vi "JSON Difference.vi"() -> ()   [LabVIEW 2019]
doc: "Shows the use of JSON Difference in JSONtext."
uses:
  vi.lib/JDP Science/JSONtext/JSONtext.lvlib
panel:
  in  "Second":string="{\n    \"balance\": \"$3,124.10\",\n    \"index\": 1,\n    \"guid\": \"787c1912-662d-48b9-b395-2ad75d217224\",\n    \"isActive\": true,\n    \"_id\": \"59b53bcb02b0cb1b19bb98a8\",\n    \"latitude\": -14.331614,\n    \"longitude\": -65.032248,\n    \"tags\": [\n      \"sint\",\n      \"magna\",\n      \"laboris\",\n      \"irure\",\n      \"aliquip\",\n      \"voluptate\"\n    ],\n    \"picture\": \"http://placehold.it/32x32\",\n    \"age\": 28,\n    \"eyeColor\": \"green\",\n    \"name\": \"Brady York\",\n    \"gender\": \"male\",\n    \"company\": \"ELEMANTRA\",\n    \"email\": \"bradyyork@elemantra.com\",\n    \"phone\": \"+1 (932) 487-3511\",\n    \"address\": \"349 Amber Street, Day, Rhode Island, 8815\",\n    \"about\": \"Culpa magna magna incididunt aliquip adipisicing incididunt. Culpa ex qui aliqua aliqua sint aliqua incididunt duis. Labore consectetur in pariatur qui anim reprehenderit duis.\\r\\n\",\n    \"registered\": \"2014-10-21T08:11:24 -01:00\",\n    \"friends\": [\n      {\n        \"id\": 0,\n        \"name\": \"Magdalena Stanley\"\n      },\n      {\n        \"id\": 1,\n        \"name\": \"Gill Alvarez\"\n      },\n      {\n        \"id\": 2,\n        \"name\": \"Alston Pacheco\"\n      }\n    ],\n    \"greeting\": \"Hello, Brady York! You have 8 unread messages.\",\n    \"favoriteFruit\": \"peach\"\n  }" caption="Second (note that the ordering of elements has been changed, which is NOT a \"difference\")"
  in  "First":string="{\n    \"_id\": \"59b53bcb02b0cb1b19bb98a8\",\n    \"index\": 0,\n    \"guid\": \"787c1912-662d-48b9-b395-2ad75d217224\",\n    \"isActive\": true,\n    \"balance\": \"$3,889.42\",\n    \"picture\": \"http://placehold.it/32x32\",\n    \"age\": 28,\n    \"eyeColor\": \"green\",\n    \"name\": \"Brady York\",\n    \"gender\": \"male\",\n    \"company\": \"ELEMANTRA\",\n    \"email\": \"bradyyork@elemantra.com\",\n    \"phone\": \"+1 (932) 487-2014\",\n    \"address\": \"349 Amber Street, Day, Rhode Island, 8815\",\n    \"about\": \"Culpa magna magna incididunt aliquip adipisicing incididunt. Culpa ex qui aliqua aliqua sint aliqua incididunt duis. Labore consectetur in pariatur qui anim reprehenderit duis.\\r\\n\",\n    \"registered\": \"2014-10-21T08:11:24 -01:00\",\n    \"latitude\": -14.331614,\n    \"longitude\": -65.032248,\n    \"tags\": [\n      \"sint\",\n      \"magna\",\n      \"laboris\",\n      \"irure\"\n    ],\n    \"friends\": [\n      {\n        \"id\": 0,\n        \"name\": \"Magdalena Stanley\"\n      },\n      {\n        \"id\": 1,\n        \"name\": \"Gill Alvarez\"\n      }\n    ],\n    \"greeting\": \"Hello, Brady York! You have 8 unread messages.\",\n    \"favoriteFruit\": \"banana\"\n  }"
  out "<JSON> 2":string caption="Changes (Second from First)"
  out "<JSON>":string caption="Changes (First from Second)"
  # "Run this VI, then see block diagram:"
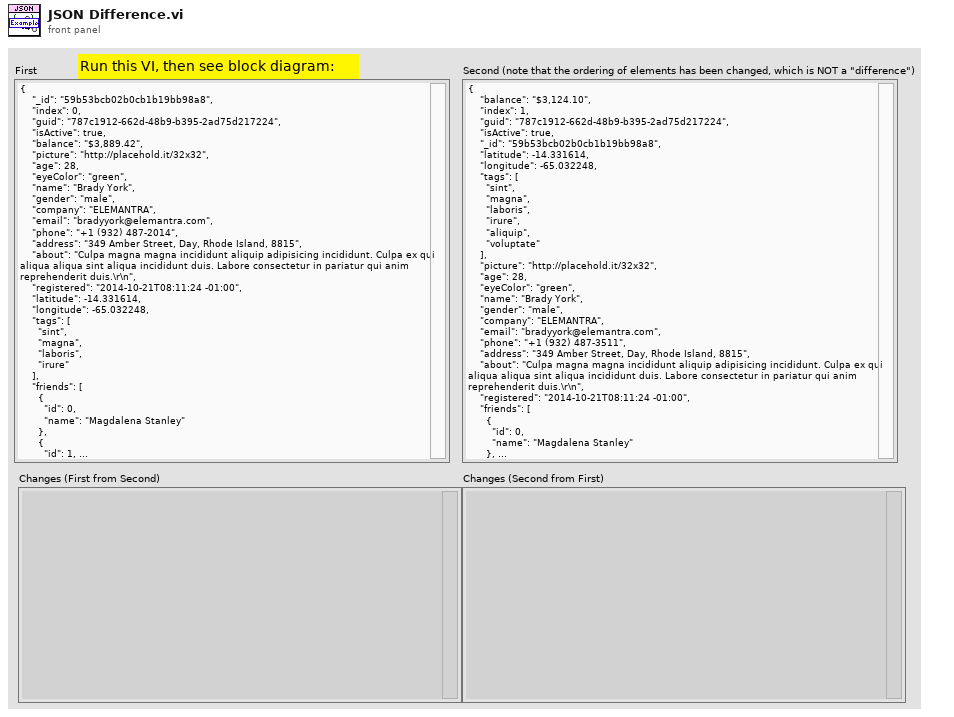
[diagram p1: front panel]
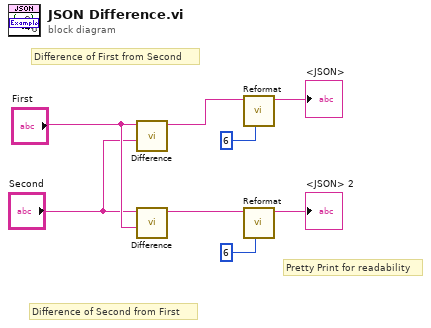
[diagram p0: block diagram]
diagram:
  # "Pretty Print for readability"
  # "Difference of Second from First"
  # "Difference of First from Second"
  n1 = call "Difference.vi"("Compare to this JSON Object"="Second", "JSON Object"="First") -> ("<JSON>"=w8:string)  [unwired: 7 in, 1 out]
  n2 = call "Difference.vi"("Compare to this JSON Object"="First", "JSON Object"="Second") -> ("<JSON>"=w3:string)  [unwired: 7 in, 1 out]
  n3 = call "Reformat.vi"("Pretty Print Levels"=6, "JSON"=w8) -> ("<JSON>"=→"<JSON>":string)  [unwired: 6 in, 3 out]
  n4 = call "Reformat.vi"("Pretty Print Levels"=6, "JSON"=w3) -> ("<JSON>"=→"<JSON> 2":string)  [unwired: 6 in, 3 out]
